vi "ALTS-2015 Read Users v1.0.vi"(8 "error in (no error)":errorcluster) -> (0 "error out":errorcluster, 3 "Users":T2(array[cluster]))   [LabVIEW 2013]
doc: "This Vi is used to get all the available user registered for the project."
uses:
  <vilib>/Utility/config.llb/NI_LVConfig.lvlib
  SLL VIs/Soliton.lib/File IO/INI/SLL Read a Section Values from INI File.llb/ALTS-2015 SLL Read a Section Values from INI File (String).vi
  Controls/ALTS-2015 User Group Enum2.ctl
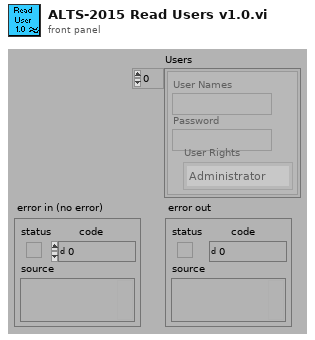
[diagram p1: front panel]
types:
  T1 = typedef "ALTS-2015 User Group Enum2.ctl" = enum16{"Administrator", "Super User", "Operator"}
  T2 = cluster{"User Names":string, "Password":string, "User Rights":T1}[]
  T3 = typedef "NI_LVConfig.lvlib/Config Data RefNum.ctl" = refnum<k1>
  T4 = typedef "ALTS-2015 User Info.ctl" = cluster{"User Name":string, "Password":string, "User Right":T1}
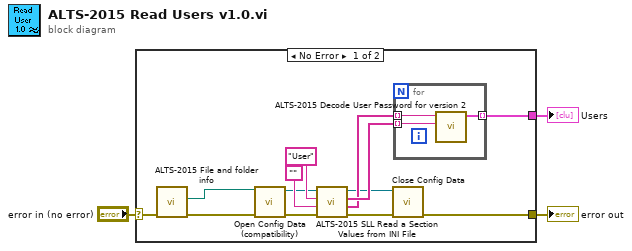
[diagram p0: block diagram]
diagram:
  n1 = case shown="No Error" "error in (no error)" {
    selector: "error in (no error)" -> [w12 w20]
    tunnel: [w5 w20] -> w3
    tunnel: [w14 _] -> w1
    frame No Error {
      n2 = call "ALTS-2015 File and folder info.vi"("error in (no error)"=w12) -> ("error out"=w9:errorcluster, "INI file path"=w4:path)  [unwired: 5 in, 4 out]
      n3 = call <vilib>:"Open Config Data (compatibility).vi"("error in (no error)"=w9, "configuration file path"=w4) -> ("error out"=w8:errorcluster, "refnum"=w10:T3)  [unwired: 7 in, 1 out]
      n4 = call-poly "ALTS-2015 SLL Read a Section Values from INI File.vi"("error in (no error)"=w8, "Default value"="", "Section"="User", "Refnum in"=w10) -> ("error out"=w6:errorcluster, "Key Names"=w11:string[], "Key Values"=w15:string[], "Refnum out"=w7:T3)  [unwired: 4 in]
      n5 = call <vilib>:"Close Config Data.vi"("error in (no error)"=w6, "refnum"=w7) -> ("error out"=w5:errorcluster)  [unwired: 8 in, 1 out]
      n6 = for {
        tunnel: w15 -> [w17] mode=indexing
        tunnel: w11 -> [w18] mode=indexing
        tunnel: [w19] -> w14 mode=indexing
        n7 = call "ALTS-2015 Decode User Password for version 2.vi"("User Value"=w17, "User Name"=w18) -> ("User Info"=w19:T4)  [unwired: 9 in]
      }
    }
    frame Error {
    }
  }
  "error out" <- w3
  "Users" <- w1
